vi "0007_FireEveryFifteenthfMonth.vi"(8 "error in (no error)":errorcluster) -> (0 "error out":errorcluster)   [LabVIEW 2013]
uses:
  <vilib>/addons/_JKI Toolkits/Caraya/classes/Assert/Assert True.vi
  <vilib>/addons/_JKI Toolkits/Caraya/classes/Test/Test.lvclass
  <vilib>/addons/_JKI Toolkits/Caraya/classes/Assert/Assert.lvclass
  source/openCron.lvlib
panel:
  out "Occurences":timestamp[](array[timestamp])
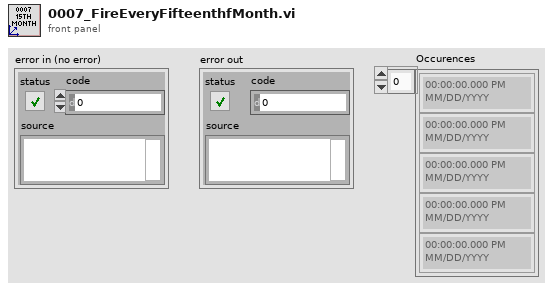
[diagram p1: front panel]
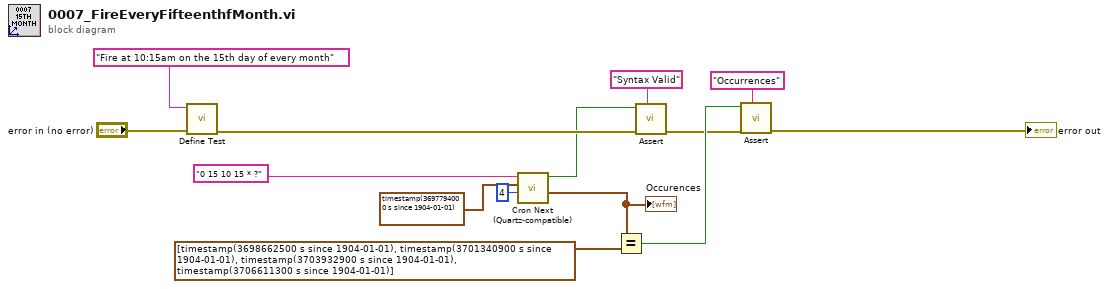
[diagram p0: block diagram]
diagram:
  n1 = call <vilib>:"Define Test.vi"("error in (no error)"="error in (no error)", "Label (VI Title)"="Fire at 10:15am on the 15th day of every month") -> ("error out"=w11:errorcluster)  [unwired: 9 in]
  n2 = call "Cron Next (Quartz-compatible).vi"("Nb Occurences (min: 1)"=u16 4, "Reference timestamp (Now)"=timestamp(3697794000 s since 1904-01-01) ("y"), "Cron Expression"="0 15 10 15 * ?" ("Expression")) -> ("Occurences"=w7:timestamp[], "syntax valid?"=w8:bool)  [unwired: 6 in, 1 out]
  "Occurences" <- w7
  n3 = Equal?(x=w7, y=timestamp[] [timestamp(3698662500 s since 1904-01-01), timestamp(3701340900 s since 1904-01-01), timestamp(3703932900 s since 1904-01-01), timestamp(3706611300 s since 1904-01-01)]) -> (x = y?=w10:bool)
  n4 = call-poly <vilib>:"Assert.vi"("Label"="Syntax Valid" ("Label (VI Title)"), "error in (no error)"=w11, "True?"=w8) -> ("error out"=w9:errorcluster)  [unwired: 8 in]
  n5 = call-poly <vilib>:"Assert.vi"("Label"="Occurrences" ("Label (VI Title)"), "error in (no error)"=w9, "True?"=w10) -> ("error out"=→"error out":errorcluster)  [unwired: 8 in]
